vi "Update terminal.vi"(11 "VI in":refnum<vi>) -> (0 "error out":errorcluster, 2 "change?":bool)   [LabVIEW 2019]
uses:
  <vilib>/Utility/traverseref.llb/TRef TravTarget.ctl
  <vilib>/numeric/LVNumericRepresentation.ctl
  <vilib>/Utility/traverseref.llb/VI Scripting - Traverse.lvlib
panel:
  in  "error in (no error)":errorcluster
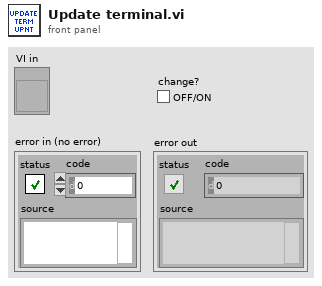
[diagram p1: front panel]
types:
  T1 = typedef "TRef TravTarget.ctl" = enum16{"FP", "BD", "Other"}
  T2 = typedef "LVNumericRepresentation.ctl" = enum32{"Extended Precision", "Double Precision", "Single Precision", "Long", "Word", "Byte", "Unsigned Long", "Unsigned Word", "Unsigned Byte", "Complex Extended", "Complex Double", "Complex Single", "Quad", "Unsigned Quad", "Fixed-Point"}
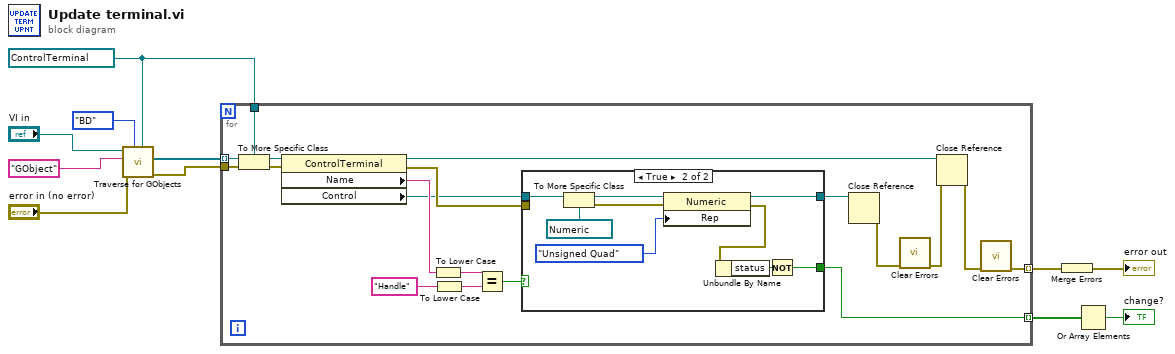
[diagram p0: block diagram]
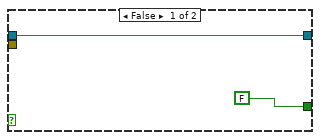
[diagram p2: hidden frame]
diagram:
  w8 = refnum<vi> refnum ("Other Refnum")
  n1 = call <vilib>:"Traverse for GObjects.vi"("Other Refnum"=w8, "Traverse Target"=TRef_TravTarget."BD", "error in (no error)"="error in (no error)", "Class Name"="GObject", "VI Refnum"="VI in") -> ("error out"=w7:errorcluster, "References"=w10:refnum<vi>[])  [unwired: 3 in, 2 out]
  n2 = for {
    tunnel: w10 -> [w28] mode=indexing
    tunnel: w8 -> [w30]
    tunnel: w7 -> [w21]
    tunnel: [w12] -> w5 mode=indexing
    tunnel: [w16] -> w3 mode=indexing
    n3 = To More Specific Class(target class=w30, reference=w28, error in=w21) -> (specific class reference=w29:refnum<vi>, error out=w22:errorcluster)
    n4 = property class="ControlTerminal"(reference=w29, error in=w22) -> (reference out=w13:refnum<vi>, error out=w19:errorcluster, "Name"=w27:string, "Control"=w18:refnum<vi>)
    n5 = To Lower Case(string=w27) -> (all lower case string=w25:string)
    n6 = To Lower Case(string="Handle" ("y")) -> (all lower case string=w24:string)
    n7 = Equal?(x=w25, y=w24) -> (x = y?=w23:bool)
    n8 = case shown="True" w23 {
      tunnel: w18 -> [w32 w40]
      tunnel: [w32 w37] -> w20
      tunnel: [FALSE w33] -> w12
      tunnel: w19 -> [_ _]
      frame False {
      }
      frame True {
        n9 = To More Specific Class(target class=refnum<vi> refnum ("Other Refnum"), reference=w40) -> (specific class reference=w39:refnum<vi>, error out=w36:errorcluster)  [unwired: 1 in]
        n10 = property class="Numeric"(reference=w39, error in=w36, "Rep"=LVNumericRepresentation."Unsigned Quad" ("Representation")) -> (reference out=w37:refnum<vi>, error out=w34:errorcluster)
        n11 = Unbundle By Name(w34) -> ("status"=w35:bool)
        n12 = Not(x=w35) -> (.not. x?=w33:bool)
      }
    }
    n13 = Close Reference(reference=w20) -> (error out=w15:errorcluster)  [unwired: 1 in]
    n14 = call <vilib>:"Clear Errors.vi"("error in (no error)"=w15) -> ("error out"=w14:errorcluster)  [unwired: 5 in, 1 out]
    n15 = Close Reference(reference=w13, error in (no error)=w14) -> (error out=w17:errorcluster)
    n16 = call <vilib>:"Clear Errors.vi"("error in (no error)"=w17) -> ("error out"=w16:errorcluster)  [unwired: 5 in, 1 out]
  }
  n17 = Merge Errors(w3) -> (→"error out":errorcluster)
  n18 = Or Array Elements(Boolean array=w5) -> (logical OR=→"change?":bool)
